vi "ApplyPersistentData.vi"(8 "error in (no error)":errorcluster, 10 "PersistentData":T1 {"RecircPumpFlow"."Recirc Pump Flow Set - R6" min=0.0 max=20.0; "RecircPumpFlow"."Recirc Pump Flow Set - R5" min=0.0 max=20.0; "RecircPumpFlow"."Recirc Pump Flow Set - R4" min=0.0 max=20.0; "RecircPumpFlow"."Recirc Pump Flow Set - R3" min=0.0 max=20.0; "RecircPumpFlow"."Recirc Pump Flow Set - R2" min=0.0 max=20.0; "RecircPumpFlow"."Recirc Pump Flow Set - R1" min=0.0 max=20.0; "MiniscusPressure"."Meniscus Pressure Set - R6" min=0.0 max=20.0; "MiniscusPressure"."Meniscus Pressure Set - R5" min=0.0 max=20.0; "MiniscusPressure"."Meniscus Pressure Set - R4" min=0.0 max=20.0; "MiniscusPressure"."Meniscus Pressure Set - R3" min=0.0 max=20.0; "MiniscusPressure"."Meniscus Pressure Set - R2" min=0.0 max=20.0; "MiniscusPressure"."Meniscus Pressure Set - R1" min=0.0 max=20.0; "Meniscus Vac Pump Speed" min=0.0 max=100.0}, 11 "TopLevel in":refnum<class "TopLevel.lvclass">) -> (0 "error out":errorcluster, 3 "TopLevel out":refnum<class "TopLevel.lvclass">)   [LabVIEW 2022 SP3, in "TopLevel.lvclass"]
uses:
  TopLevel.lvclass
  Common/Controls/PersistentData--Cluster.ctl
  Typedefs/API Command Enum.ctl
  Typedefs/PrinterHeads--Enum.ctl
  IO/Typedefs/ICP1-AO Channel Names.ctl
  Typedefs/API Command Cluster.ctl
  GIS Printer/GIS Printer.lvclass/GIS Printer.ctl
  GIS Printer/Methods/Variant_To_DVR.vi
  GIS Printer/GIS Printer.lvclass
  DAQWFE/LV_Source/Subsystems/DAQ/DAQ.lvclass
  IO/IO.lvclass
  IO/Typedefs/ICP2-AO Channel Names.ctl
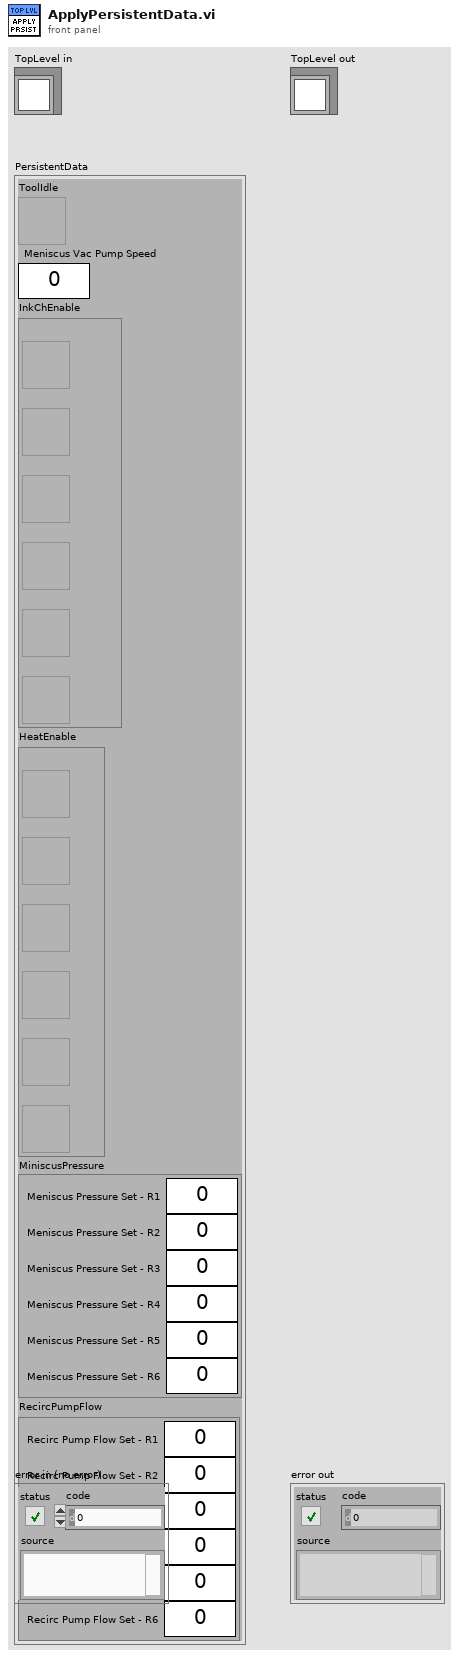
[diagram p1: front panel]
types:
  T1 = typedef "PersistentData--Cluster.ctl" = cluster{"ToolIdle":bool, "Meniscus Vac Pump Speed":dbl, "InkChEnable":cluster{"Enable Ink Ch-1":bool, "Enable Ink Ch-2":bool, "Enable Ink Ch-3":bool, "Enable Ink Ch-4":bool, "Enable Ink Ch-5":bool, "Enable Ink Ch-6":bool}, "HeatEnable":cluster{"Heater-1 Off":bool, "Heater-2 Off":bool, "Heater-3 Off":bool, "Heater-4 Off":bool, "Heater-5 Off":bool, "Heater-6 Off":bool}, "MiniscusPressure":cluster{"Meniscus Pressure Set - R1":dbl, "Meniscus Pressure Set - R2":dbl, "Meniscus Pressure Set - R3":dbl, "Meniscus Pressure Set - R4":dbl, "Meniscus Pressure Set - R5":dbl, "Meniscus Pressure Set - R6":dbl}, "RecircPumpFlow":cluster{"Recirc Pump Flow Set - R1":dbl, "Recirc Pump Flow Set - R2":dbl, "Recirc Pump Flow Set - R3":dbl, "Recirc Pump Flow Set - R4":dbl, "Recirc Pump Flow Set - R5":dbl, "Recirc Pump Flow Set - R6":dbl}}
  T2 = typedef "IO.lvclass/ICP1-AO Channel Names.ctl" = enum16{"None", "Meniscus Pressure Set - R1", "Meniscus Pressure Set - R2", "Meniscus Pressure Set - R3", "Meniscus Pressure Set - R4", "Meniscus Pressure Set - R5", "Meniscus Pressure Set - R6", "Meniscus Vac Pump Speed"}
  T3 = typedef "PrinterHeads--Enum.ctl" = enum16{"-1", "1", "2", "3", "4", "5", "6"}
  T4 = typedef "TopLevel.lvclass/API Command Enum.ctl" = enum16{"Execute Printer Commands", "Pre Purge", "Enable Ink Ch-1", "Enable Ink Ch-2", "Enable Ink Ch-3", "Enable Ink Ch-4", "Enable Ink Ch-5", "Enable Ink Ch-6", "Disable Ink Ch-1", "Disable Ink Ch-2", "Disable Ink Ch-3", "Disable Ink Ch-4", "Disable Ink Ch-5", "Disable Ink Ch-6", "ExecuteIdlePrintCycle", "StopIdlePrintCycle", "Abort", "LoadDLP2GUIConfig", "SaveDLP2GUIConfig", "PrimingMode", "SetHeadTemperature", "EnableHead", "EnableHeadHeat", "SetSystemMode", "HeadPrint", "AbortAll", "Send Printer String", "WriteInitXML"}
  T5 = typedef "DLPConfig_Initialization.ctl" = cluster{"PrinterInitialization":cluster{"Printer":cluster{"#attributes":cluster{"Name":string}}, "VacPumpSet":cluster{"#attributes":cluster{"VacPumpEnable":bool, "VacPumpSpeed":dbl}}, "HIBEnable":cluster{"#attributes":cluster{"HIB1Enable":bool, "HIB2Enable":bool, "HIB3Enable":bool, "HIB4Enable":bool, "HIB5Enable":bool, "HIB6Enable":bool}}, "PrinterCompensation":T6}, "HeadSet":cluster{"HeadProperties":T7[]}, "InkSet":cluster{"Ink":T9[]}, "Troubleshooting":cluster{"PMBLogging":cluster{"#attributes":cluster{"PMBMonitorDuringPrint":bool, "PMBMonitorDuringIdle":bool, "LogSwatheInputData":bool, "LogSwatheOutputData":bool, "LogPrintheadColourPlanes":bool, "LogPMBCommunication":bool, "LogSimulatedOutput":bool, "LogAllPMBCommunicationData":bool, "LogPMBSpace":bool, "ExtendedPMBSpaceLogging":bool, "LogPMBWriteSpeed":bool, "LogUsbRetries":bool}}, "HIBLogging":cluster{"#attributes":cluster{"HIBMonitoringDuringPrint":bool, "HIBMonitoringLog":bool}}}}
  T6 = typedef "DLP2_PrinterCompensationProperties.ctl" = cluster{"#attributes":cluster{"AppName":string, "PrintWeightMultiplier":dbl, "Rotation":bool, "Driver":string, "Server":string, "Database":string, "User":string, "Password":string}}
  T7 = typedef "DLP2_PrinterHeadProperties.ctl" = cluster{"#attributes":T8}
  T8 = typedef "DLPConfig)Init_HeadPropertyAttr--Cluster.ctl" = cluster{"HeadNumber":u8, "Material":string, "HeadLocalX":dbl, "HeadLocalY":dbl, "HeadRotationAngle":dbl, "VH2L_Hi":dbl, "VH2R_Hi":dbl, "VH1LA_Hi":dbl, "VH1LB_Hi":dbl, "VH1RA_Hi":dbl, "VH1RB_Hi":dbl, "VH2L_Lo":dbl, "VH2R_Lo":dbl, "VH1LA_Lo":dbl, "VH1LB_Lo":dbl, "VH1RA_Lo":dbl, "VH1RB_Lo":dbl}
  T9 = typedef "DLP2_PrinterMaterialProperties.ctl" = cluster{"#attributes":cluster{"InkType":string, "ColorPlane":string, "PrePrintPurge":bool, "PurgeTime":dbl, "PurgeCount":i32, "Density":dbl, "NumberofDrops":i32, "PrintWeight":dbl, "PrintheadPrime":bool}, "Idle":T10, "Process":T11}
  T10 = typedef "InkIdleNodeConfigXML--Cluster.ctl" = cluster{"ShortIdle":cluster{"#attributes":cluster{"Heat":dbl, "Meniscus":dbl, "Recirculation":bool}}, "LongIdle":cluster{"#attributes":cluster{"Heat":dbl, "Meniscus":dbl, "Recirculation":bool}}}
  T11 = typedef "InkProcessNodeConfigXML--Cluster.ctl" = cluster{"C30_Process":cluster{"#attributes":cluster{"Heat":dbl, "Meniscus":dbl, "Recirculation":bool, "ColorPlane":string}}, "S30_Process":cluster{"#attributes":cluster{"Heat":dbl, "Meniscus":dbl, "Recirculation":bool, "ColorPlane":string}}}
  T12 = cluster{"Recirc Pump Flow Set - R1":dbl, "Recirc Pump Flow Set - R2":dbl, "Recirc Pump Flow Set - R3":dbl, "Recirc Pump Flow Set - R4":dbl, "Recirc Pump Flow Set - R5":dbl, "Recirc Pump Flow Set - R6":dbl}
  T13 = cluster{"Meniscus Pressure Set - R1":dbl, "Meniscus Pressure Set - R2":dbl, "Meniscus Pressure Set - R3":dbl, "Meniscus Pressure Set - R4":dbl, "Meniscus Pressure Set - R5":dbl, "Meniscus Pressure Set - R6":dbl}
  T14 = cluster{"Heater-1 Off":bool, "Heater-2 Off":bool, "Heater-3 Off":bool, "Heater-4 Off":bool, "Heater-5 Off":bool, "Heater-6 Off":bool}
  T15 = cluster{"Enable Ink Ch-1":bool, "Enable Ink Ch-2":bool, "Enable Ink Ch-3":bool, "Enable Ink Ch-4":bool, "Enable Ink Ch-5":bool, "Enable Ink Ch-6":bool}
  T16 = cluster{"HIB1Enable":bool, "HIB2Enable":bool, "HIB3Enable":bool, "HIB4Enable":bool, "HIB5Enable":bool, "HIB6Enable":bool}
  T17 = typedef "TopLevel.lvclass/API Command Cluster.ctl" = cluster{"Command":T4, "Arguments":string, "Data":variant}
  T18 = typedef "GIS Status--Cluster.ctl" = cluster{"HeadEnabled":bool, "SpitEnabled":bool, "HeaterEnabled":bool, "TargetTemperature":dbl, "CurrentTemperature":dbl}
  T19 = typedef "IO.lvclass/ICP2-AO Channel Names.ctl" = enum16{"None", "Recirc Pump Flow Set - R1", "Recirc Pump Flow Set - R2", "Recirc Pump Flow Set - R3", "Recirc Pump Flow Set - R4", "Recirc Pump Flow Set - R5", "Recirc Pump Flow Set - R6"}
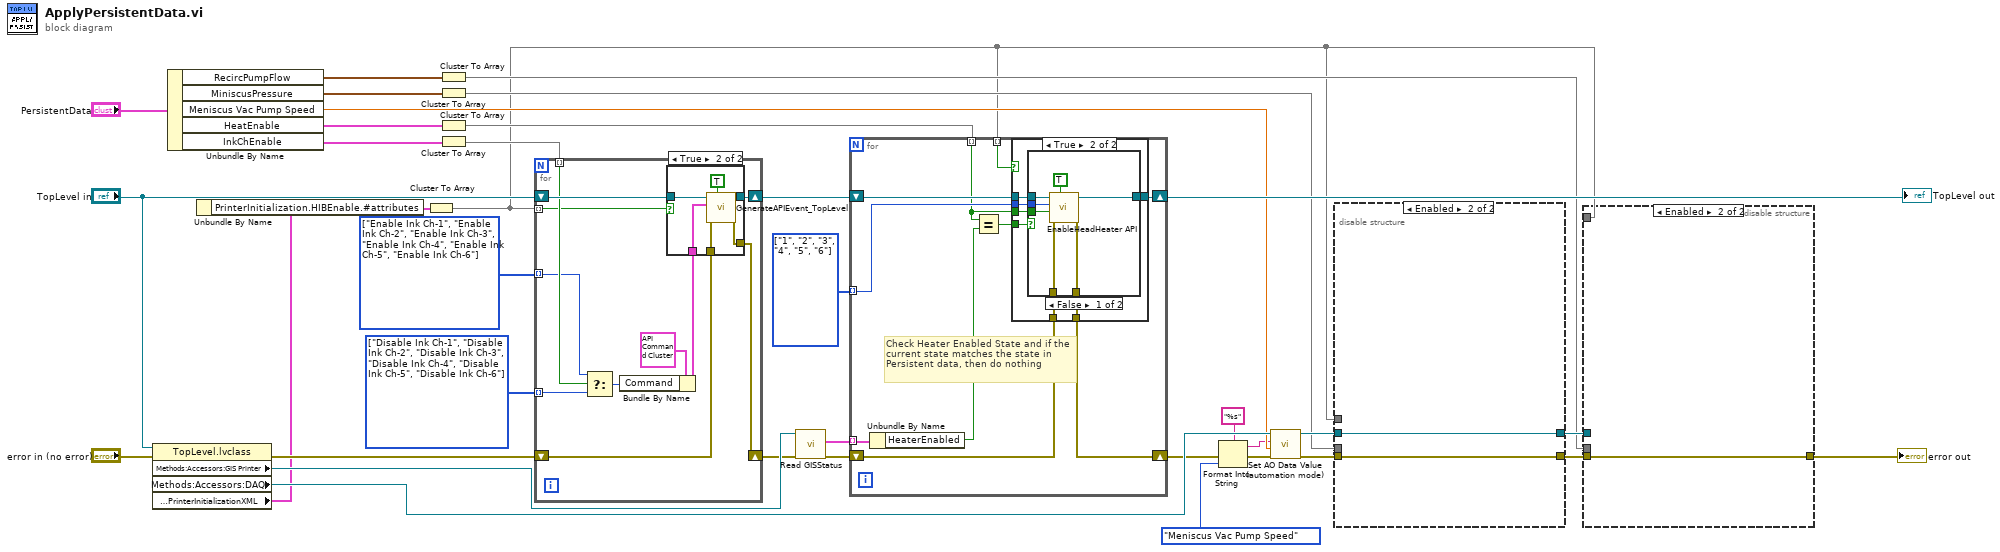
[diagram p0: block diagram]
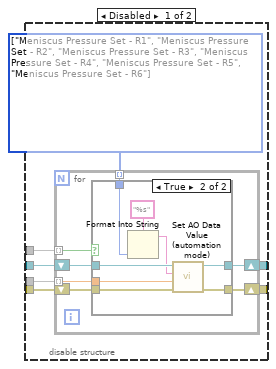
[diagram p2: hidden frame]
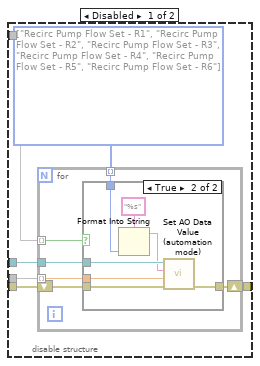
[diagram p4: hidden frame]
diagram:
  w29 = T3[] [enum."1", enum."2", enum."3", enum."4", enum."5", enum."6"] items=["-1", "1", "2", "3", "4", "5", "6"] ("Heater Enable.Head")
  w34 = T4[] [enum."Disable Ink Ch-1", enum."Disable Ink Ch-2", enum."Disable Ink Ch-3", enum."Disable Ink Ch-4", enum."Disable Ink Ch-5", enum."Disable Ink Ch-6"] items=["Execute Printer Commands", "Pre Purge", "Enable Ink Ch-1", "Enable Ink Ch-2", "Enable Ink Ch-3", "Enable Ink Ch-4", "Enable Ink Ch-5", "Enable Ink Ch-6", "Disable Ink Ch-1", "Disable Ink Ch-2", "Disable Ink Ch-3", "Disable Ink Ch-4", "Disable Ink Ch-5", "Disable Ink Ch-6", "ExecuteIdlePrintCycle", "StopIdlePrintCycle", "Abort", "LoadDLP2GUIConfig", "SaveDLP2GUIConfig", "PrimingMode", "SetHeadTemperature", "EnableHead", "EnableHeadHeat", "SetSystemMode", "HeadPrint", "AbortAll", "Send Printer String", "WriteInitXML"]
  w33 = T4[] [enum."Enable Ink Ch-1", enum."Enable Ink Ch-2", enum."Enable Ink Ch-3", enum."Enable Ink Ch-4", enum."Enable Ink Ch-5", enum."Enable Ink Ch-6"] items=["Execute Printer Commands", "Pre Purge", "Enable Ink Ch-1", "Enable Ink Ch-2", "Enable Ink Ch-3", "Enable Ink Ch-4", "Enable Ink Ch-5", "Enable Ink Ch-6", "Disable Ink Ch-1", "Disable Ink Ch-2", "Disable Ink Ch-3", "Disable Ink Ch-4", "Disable Ink Ch-5", "Disable Ink Ch-6", "ExecuteIdlePrintCycle", "StopIdlePrintCycle", "Abort", "LoadDLP2GUIConfig", "SaveDLP2GUIConfig", "PrimingMode", "SetHeadTemperature", "EnableHead", "EnableHeadHeat", "SetSystemMode", "HeadPrint", "AbortAll", "Send Printer String", "WriteInitXML"]
  n1 = property class="TopLevel.lvclass"(reference="TopLevel in", error in="error in (no error)") -> (error out=w24:errorcluster, "Methods:Accessors:GIS Printer"=w23:refnum<class "GIS Printer.lvclass">, "Methods:Accessors:DAQ"=w19:refnum<class "DAQ.lvclass">, "Methods:Accessors:PrinterInitializationXML"=w5:T5)  [unwired: 1 out]
  n2 = Unbundle By Name("PersistentData") -> ("RecircPumpFlow"=w7:T12, "MiniscusPressure"=w12:T13, "Meniscus Vac Pump Speed"=w18:dbl, "HeatEnable"=w28:T14, "InkChEnable"=w36:T15)
  n3 = Unbundle By Name(w5) -> ("PrinterInitialization.HIBEnable.#attributes"=w4:T16)
  n4 = Cluster To Array(cluster=w4) -> (array=w3:bool[])
  n5 = Cluster To Array(cluster=w7) -> (array=w6:dbl[])
  n6 = Cluster To Array(cluster=w12) -> (array=w11:dbl[])
  n7 = Cluster To Array(cluster=w28) -> (array=w27:bool[])
  n8 = Cluster To Array(cluster=w36) -> (array=w32:bool[])
  n9 = for {
    shift-right: [w44] -> w31
    shift-left: "TopLevel in" -> [w45]
    tunnel: w32 -> [w43] mode=indexing
    tunnel: w33 -> [w42] mode=indexing
    tunnel: w34 -> [w41] mode=indexing
    shift-right: [w38] -> w22
    shift-left: w24 -> [w39]
    tunnel: w3 -> [w37] mode=indexing
    n10 = Select(t=w42, s=w43, f=w41) -> (s? t:f=w40:T4)
    n11 = Bundle By Name(cluster=T17 {"Command"=enum."Execute Printer Commands", "Arguments"="", "Data"=variant} ("API Command Cluster"), "Command"=w40) -> (w46:T17)
    n12 = case shown="True" w37 {
      tunnel: w46 -> [_ w55]
      tunnel: w45 -> [w49 w54]
      tunnel: [w49 w53] -> w44
      tunnel: w39 -> [w48 w52]
      tunnel: [w48 w51] -> w38
      frame False {
      }
      frame True {
        n13 = call-dynamic "GenerateAPIEvent_TopLevel.vi"("Wait (F)"=TRUE, "error in (no error)"=w52, "API Command Cluster"=w55, "TopLevel in"=w54) -> ("error out"=w51:errorcluster, "TopLevel out"=w53:refnum<class "TopLevel.lvclass">)  [unwired: 6 in]
      }
    }
  }
  n14 = call "Read GISStatus.vi"("error in (no error)"=w22, "GIS Printer in"=w23) -> ("error out"=w21:errorcluster, "GISHeadStatus"=w20:T18[])  [unwired: 7 in, 1 out]
  n15 = for {
    shift-right: [w64] -> w30
    shift-left: w31 -> [w65]
    shift-right: [w62] -> w2
    shift-left: w21 -> [w63]
    tunnel: w29 -> [w61] mode=indexing
    tunnel: w27 -> [w57] mode=indexing
    tunnel: w20 -> [w60] mode=indexing
    tunnel: w3 -> [w56] mode=indexing
    # "Check Heater Enabled State and if the current state matches the state in Persistent data, then do nothing"
    n16 = Unbundle By Name(w60) -> ("HeaterEnabled"=w59:bool)
    n17 = Equal?(x=w57, y=w59) -> (x = y?=w58:bool)
    n18 = case shown="True" w56 {
      tunnel: w65 -> [w67 w74]
      tunnel: [w67 w73] -> w64
      tunnel: w63 -> [w66 w72]
      tunnel: [w66 w71] -> w62
      tunnel: w61 -> [_ w70]
      tunnel: w58 -> [_ w69]
      tunnel: w57 -> [_ w68]
      frame False {
      }
      frame True {
        n19 = case shown="False" w69 {
          tunnel: w74 -> [w81 w82]
          tunnel: [w80 w82] -> w73
          tunnel: w72 -> [w79 w83]
          tunnel: [w78 w83] -> w71
          tunnel: w70 -> [w77 _]
          tunnel: w68 -> [w76 _]
          frame False {
            n20 = call-dynamic "EnableHeadHeater API.vi"("Wait (F)"=TRUE, "error in (no error)"=w79, "Enable"=w76, "Head"=w77, "TopLevel in"=w81) -> ("error out"=w78:errorcluster, "TopLevel out"=w80:refnum<class "TopLevel.lvclass">)  [unwired: 5 in]
          }
          frame True {
          }
        }
      }
    }
  }
  "TopLevel out" <- w30
  n21 = Format Into String(format string="%s", error in=w2, ICP1-AO_Channel_Names."Meniscus Vac Pump Speed" ("AO Channel")) -> (resulting string=w15:string, error out=w1:errorcluster)  [unwired: 1 in]
  n22 = call "Set AO Data Value (automation mode).vi"("error in (no error)"=w1, "Value"=w18, "AO IOName"=w15, "DAQ"=w19) -> ("error out"=w14:errorcluster, "DAQ"=w13:refnum<class "DAQ.lvclass">)  [unwired: 6 in]
  n23 = disable-structure shown="Enabled" {
    disable-tunnel: w14 -> [w90 w109]
    disable-tunnel: w13 -> [w89 w108]
    disable-tunnel: w11 -> [w87 _]
    disable-tunnel: [w86 w109] -> w10
    disable-tunnel: [w85 w108] -> w8
    disable-tunnel: w3 -> [w84 _]
    frame Disabled {
      w88 = T2[] [enum."Meniscus Pressure Set - R1", enum."Meniscus Pressure Set - R2", enum."Meniscus Pressure Set - R3", enum."Meniscus Pressure Set - R4", enum."Meniscus Pressure Set - R5", enum."Meniscus Pressure Set - R6"] items=["None", "Meniscus Pressure Set - R1", "Meniscus Pressure Set - R2", "Meniscus Pressure Set - R3", "Meniscus Pressure Set - R4", "Meniscus Pressure Set - R5", "Meniscus Pressure Set - R6", "Meniscus Vac Pump Speed"] ("AO Channel")
      n24 = for {
        shift-right: [w96] -> w86
        shift-left: w90 -> [w97]
        tunnel: w88 -> [w94] mode=indexing
        tunnel: w87 -> [w93] mode=indexing
        shift-right: [w92] -> w85
        shift-left: w89 -> [w95]
        tunnel: w84 -> [w91] mode=indexing
        n25 = case shown="True" w91 {
          tunnel: w97 -> [w98 w106]
          tunnel: [w98 w105] -> w96
          tunnel: w95 -> [w99 w104]
          tunnel: w94 -> [_ w102]
          tunnel: w93 -> [_ w101]
          tunnel: [w99 w100] -> w92
          frame False {
          }
          frame True {
            n26 = Format Into String(format string="%s", w102) -> (resulting string=w103:string)  [unwired: 2 in, 1 out]
            n27 = call "Set AO Data Value (automation mode).vi"("error in (no error)"=w106, "Value"=w101, "AO IOName"=w103, "DAQ"=w104) -> ("error out"=w105:errorcluster, "DAQ"=w100:refnum<class "DAQ.lvclass">)  [unwired: 6 in]
          }
        }
      }
    }
    frame Enabled {
    }
  }
  n28 = disable-structure shown="Enabled" {
    disable-tunnel: w10 -> [w115 w130]
    disable-tunnel: [w114 w130] -> w9
    disable-tunnel: w8 -> [w113 _]
    disable-tunnel: w6 -> [w111 _]
    disable-tunnel: w3 -> [w110 _]
    frame Disabled {
      w112 = T19[] [enum."Recirc Pump Flow Set - R1", enum."Recirc Pump Flow Set - R2", enum."Recirc Pump Flow Set - R3", enum."Recirc Pump Flow Set - R4", enum."Recirc Pump Flow Set - R5", enum."Recirc Pump Flow Set - R6"] items=["None", "Recirc Pump Flow Set - R1", "Recirc Pump Flow Set - R2", "Recirc Pump Flow Set - R3", "Recirc Pump Flow Set - R4", "Recirc Pump Flow Set - R5", "Recirc Pump Flow Set - R6"] ("AO Channel")
      n29 = for {
        shift-right: [w120] -> w114
        shift-left: w115 -> [w121]
        tunnel: w113 -> [w119]
        tunnel: w112 -> [w118] mode=indexing
        tunnel: w111 -> [w117] mode=indexing
        tunnel: w110 -> [w116] mode=indexing
        n30 = case shown="True" w116 {
          tunnel: w121 -> [w122 w128]
          tunnel: [w122 w127] -> w120
          tunnel: w119 -> [_ w126]
          tunnel: w118 -> [_ w124]
          tunnel: w117 -> [_ w123]
          frame False {
          }
          frame True {
            n31 = Format Into String(format string="%s", w124) -> (resulting string=w125:string)  [unwired: 2 in, 1 out]
            n32 = call "Set AO Data Value (automation mode).vi"("error in (no error)"=w128, "Value"=w123, "AO IOName"=w125, "DAQ"=w126) -> ("error out"=w127:errorcluster)  [unwired: 6 in, 1 out]
          }
        }
      }
    }
    frame Enabled {
    }
  }
  "error out" <- w9
